vi "half adder 1.vi"(10 "B":bool, 11 "A":bool) -> (2 "Boolean":bool, 3 "Boolean 2":bool)   [LabVIEW 2018]
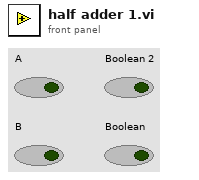
[diagram p1: front panel]
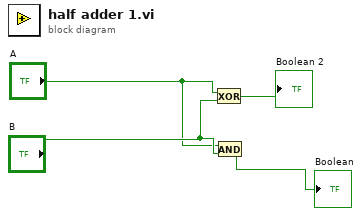
[diagram p0: block diagram]
diagram:
  n1 = Exclusive Or(1:"B", 2:"A") -> (0:→"Boolean 2":bool)
  n2 = And(x="A", y="B") -> (x .and. y?=→"Boolean":bool)
